vi "MCL_calibration.vi"() -> ()   [LabVIEW 2015]
uses:
  <vilib>/rvi/Emulation/niFpgaGetClockAttributes.vi
  <vilib>/rvi/Emulation/niFpgaSctlEmulationGetInTimedLoop.vi
  <vilib>/rvi/Emulation/niFpgaEmulationReportErrorSimple.vi
  <vilib>/rvi/eio/common/nirviEmuTemplateMethod_errors.vi
  <vilib>/rvi/Emulation/niFpgaCriticalErrorInLSC.vi
  <vilib>/eio/EIONode/EIONode.xnode
panel:
  in  "stop":bool
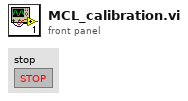
[diagram p1: front panel]
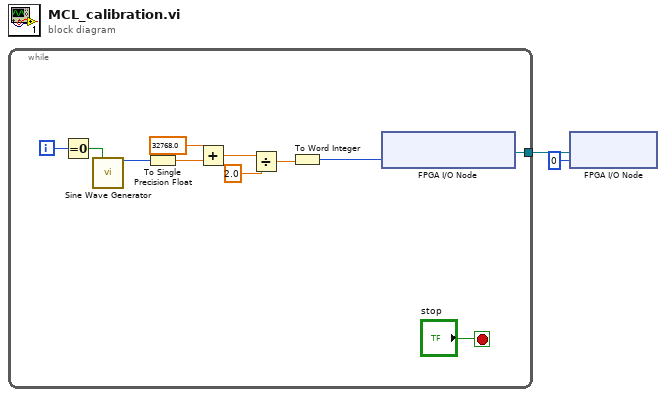
[diagram p0: block diagram]
diagram:
  n1 = while {
    tunnel: [w3] -> w2
    i -> [w12]
    stop <- "stop" stop-if-true
    n2 = Equal To 0?(x=w12) -> (x = 0?=w11:bool)
    n3 = call "Sine Wave Generator"("reset"=w11) -> ("sine out"=w5:i16)  [unwired: 14 in]
    n4 = To Single Precision Float(number=w5) -> (single precision float=w10:sgl)
    n5 = Add(x=sgl 32768.0, y=w10) -> (x+y=w4:sgl)
    n6 = Divide(x=w4, y=sgl 2.0) -> (x/y=w7:sgl)
    n7 = To Word Integer(number=w7) -> (16bit integer=w6:i16)
    n8 = xnode "FPGA I/O Node"("Connector0/AO0"=w6) -> ("FPGA I/O Out"=w3:refnum<k21>)  [unwired: 1 in]
  }
  n9 = xnode "FPGA I/O Node"("I/O Item"=i16 0, "FPGA I/O In"=w2) -> ()  [unwired: 1 out]
